vi "Add When Icon Overlay.vi"(8 "error in (no error)":errorcluster, 11 "VI in":refnum<vi>) -> (0 "error out":errorcluster, 3 "VI out":refnum<vi>)   [LabVIEW 2020, in "Mock Class Generator.lvclass"]
uses:
  Mock Class Generator.lvclass
  <vilib>/LabVIEW Icon API/API_User Layer Data.ctl
  <vilib>/Utility/miscctls.llb/LVPoint32TypeDef.ctl
  <vilib>/picture/picture.llb/imagedata.ctl
  Mock Class Generator.lvclass/Mock Class Generator.ctl
  <vilib>/LabVIEW Icon API/LabVIEW Icon API.lvlib
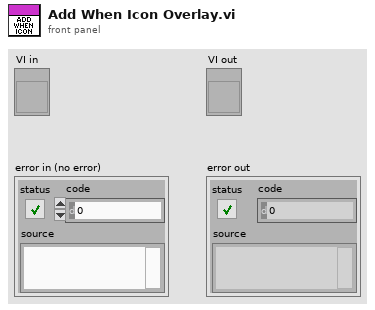
[diagram p1: front panel]
types:
  T1 = typedef "LabVIEW Icon API.lvlib/API_User Layer Data.ctl" = cluster{"Layer name":string, "Origin":T2, "Icon image data":T3}
  T2 = typedef "LVPoint32TypeDef.ctl" = cluster{"Horizontal":i32, "Vertical":i32}
  T3 = typedef "imagedata.ctl" = cluster{"image type":i32, "image depth":i32, "image":u8[], "mask":u8[], "colors":u32[], "Rectangle":cluster{"left":i16, "top":i16, "right":i16, "bottom":i16}}
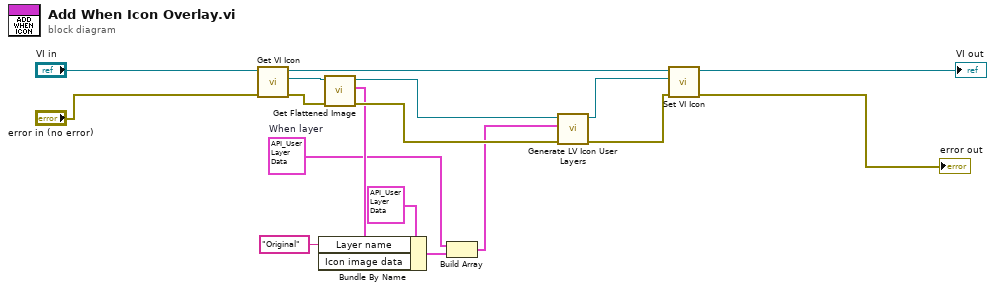
[diagram p0: block diagram]
diagram:
  w1 = T1 {"Layer name"="When", "Origin"={"Horizontal"=0, "Vertical"=0}, "Icon image data"={"image type"=0, "image depth"=24, "image"=[255, 255, 255, 255, 255, 255, 255, 255, 255, 255, 255, 255, 255, 255, 255, 255, 255, 255, 255, 255, 255, 255, 255, 255, 255, 255, 255, 255, 255, 255, 255, 255, 255, 255, 255, 255, 255, 255, 255, 255, 255, 255, 255, 255, 255, 255, 255, 255, 255, 255, 255, 255, 255, 255, 255, 255, 255, 255, 255, 255, 255, 255, 255, 255, 255, 255, 255, 255, 255, 0, 0, 0, 0, 0, 0, 255, 255, 255, 255, 255, 255, 255, 255, 255, 255, 255, 255, 255, 255, 255, 1, 1, 1, 1, 1, 1, 255, 255, 255, 255, 255, 255, 255, 255, 255, 255, 255, 255, 255, 255, 255, 255, 255, 255, 255, 255, 255, 255, 255, 255, 0, 0, 0, 0, 0, 0, 0, 0, 0, 0, 0, 0, 0, 0, 0, 0, 0, 0, 255, 255, 255, 255, 255, 255, 255, 255, 255, 1, 1, 1, 1, 1, 1, 1, 1, 1, 255, 255, 255, 255, 255, 255, 255, 255, 255, 255, 255, 255, 255, 255, 255, 255, 255, 255, 0, 0, 0, 0, 0, 0, 0, 0, 0, 255, 250, 0, 255, 250, 0, 0, 0, 0, 0, 0, 0, 0, 0, 0, 255, 255, 255, 255, 255, 255, 1, 1, 1, 1, 1, 1, 255, 250, 0, 1, 1, 1, 255, 255, 255, 255, 255, 255, 255, 255, 255, 255, 255, 255, 255, 255, 255, 0, 0, 0, 0, 0, 0, 255, 250, 0, 255, 250, 0, 255, 250, 0, 255, 250, 0, 0, 0, 0, 0, 0, 0, 255, 255, 255, 255, 255, 255, 1, 1, 1, 1, 1, 1, 255, 250, 0, 255, 250, 0, 1, 1, 1, 1, 1, 1, 255, 255, 255, 255, 255, 255, 0, 0, 0, 0, 0, 0, 255, 250, 0, 255, 250, 0, 255, 250, 0, 255, 250, 0, 255, 250, 0, 255, 250, 0, 0, 0, 0, 0, 0, 0, 255, 255, 255, 1, 1, 1, 1, 1, 1, 255, 250, 0, 255, 250, 0, 255, 250, 0, 1, 1, 1, 1, 1, 1, 255, 255, 255, 0, 0, 0, 0, 0, 0, 255, 250, 0, 255, 250, 0, 255, 250, 0, 255, 250, 0, 255, 250, 0, 255, 250, 0, 0, 0, 0, 0, 0, 0, 255, 255, 255, 1, 1, 1, 1, 1, 1, 255, 250, 0, 255, 250, 0, 255, 250, 0, 1, 1, 1, 1, 1, 1, 1, 1, 1, 255, 255, 255, 0, 0, 0, 0, 0, 0, 255, 250, 0, 255, 250, 0, 255, 250, 0, 255, 250, 0, 0, 0, 0, 0, 0, 0, 255, 255, 255, 255, 255, 255, 1, 1, 1, 1, 1, 1, 255, 250, 0, 255, 250, 0, 1, 1, 1, 1, 1, 1, 1, 1, 1, 255, 255, 255, 255, 255, 255, 0, 0, 0, 0, 0, 0, 0, 0, 0, 255, 250, 0, 255, 250, 0, 0, 0, 0, 0, 0, 0, 0, 0, 0, 255, 255, 255, 255, 255, 255, 1, 1, 1, 1, 1, 1, 255, 250, 0, 1, 1, 1, 1, 1, 1, 255, 255, 255, 255, 255, 255, 255, 255, 255, 255, 255, 255, 255, 255, 255, 0, 0, 0, 0, 0, 0, 0, 0, 0, 0, 0, 0, 0, 0, 0, 0, 0, 0, 255, 255, 255, 255, 255, 255, 255, 255, 255, 1, 1, 1, 1, 1, 1, 1, 1, 1, 1, 1, 1, 255, 255, 255, 255, 255, 255, 255, 255, 255, 255, 255, 255, 255, 255, 255, 255, 255, 255, 255, 255, 255, 255, 255, 255, 0, 0, 0, 0, 0, 0, 255, 255, 255, 255, 255, 255, 255, 255, 255, 255, 255, 255, 255, 255, 255, 1, 1, 1, 1, 1, 1, 255, 255, 255, 255, 255, 255, 255, 255, 255, 255, 255, 255, 255, 255, 255, 255, 255, 255], "mask"=[], "colors"=[], "Rectangle"={"left"=10, "top"=13, "right"=29, "bottom"=24}}}  # When layer
  n1 = call <vilib>:"Get VI Icon.vi"("error in (no error)"="error in (no error)", "VI Refnum in"="VI in") -> ("error out"=w8:errorcluster, "Icon"=w10:refnum<class "Icon.lvclass">, "VI Refnum out"=w14:refnum<vi>)  [unwired: 7 in]
  n2 = call <vilib>:"Get Flattened Image.vi"("error in (no error)"=w8, "lv_icon.lvlib:Icon.lvclass in"=w10) -> ("error out"=w7:errorcluster, "Color Image"=w5:T3, "lv_icon.lvlib:Icon.lvclass out"=w9:refnum<class "Icon.lvclass">)  [unwired: 6 in, 1 out]
  n3 = Bundle By Name(cluster=T1 {"Layer name"="", "Origin"={"Horizontal"=0, "Vertical"=0}, "Icon image data"={"image type"=0, "image depth"=0, "image"=[], "mask"=[], "colors"=[], "Rectangle"={"left"=0, "top"=0, "right"=0, "bottom"=0}}} ("appended array"), "Layer name"="Original", "Icon image data"=w5) -> (w3:T1)
  n4 = Build Array(w1, w3) -> (w2:T1[])
  n5 = call <vilib>:"Generate LV Icon User Layers.vi"("error in (no error)"=w7, "User layers"=w2, "Icon in"=w9) -> ("error out"=w11:errorcluster, "Icon out"=w12:refnum<class "Icon.lvclass">)  [unwired: 7 in]
  n6 = call <vilib>:"Set VI Icon.vi"("error in (no error)"=w11, "Icon"=w12, "VI Refnum in"=w14) -> ("error out"=→"error out":errorcluster, "VI Refnum out"=→"VI out":refnum<vi>)  [unwired: 7 in]
